vi "RL Control.vi"() -> ()   [LabVIEW 2014]
uses:
  <vilib>/express/express arith-compare/Formula/XNode/ExpressFormulaBlockNode.xnode
panel:
  in  "VARS":dbl(slide) scale=8.0..19.0
  in  "?":bool
  in  "VARS User Input":dbl
  in  "Selector Switch":bool
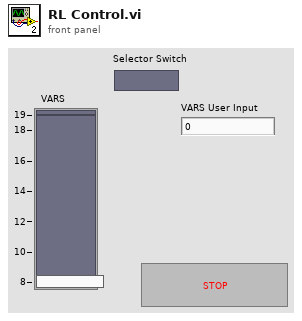
[diagram p1: front panel]
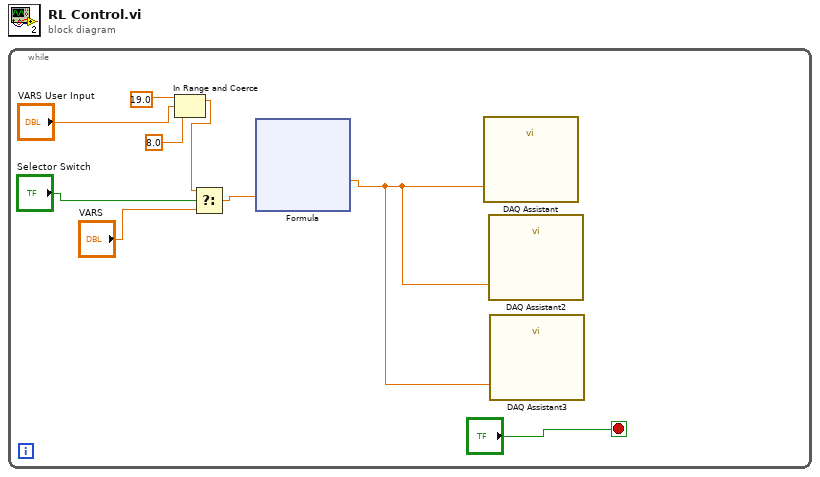
[diagram p0: block diagram]
diagram:
  n1 = while {
    stop <- "?" stop-if-true
    n2 = In Range and Coerce(upper limit=19.0, x="VARS User Input", lower limit=8.0) -> (coerced(x)=w3:dbl)  [unwired: 1 out]
    n3 = Select(t=w3, s="Selector Switch", f="VARS") -> (s? t:f=w9:dbl)
    n4 = xnode "Formula"("X"=w9) -> ("Result"=w1:dbl)  [unwired: 1 in, 1 out]
    n5 = call "DAQ Assistant"("data"=w1) -> ()  [unwired: 17 in, 2 out]
    n6 = call "DAQ Assistant2"("data"=w1) -> ()  [unwired: 17 in, 2 out]
    n7 = call "DAQ Assistant3"("data"=w1) -> ()  [unwired: 17 in, 2 out]
  }
